vi "PDF Standard Kopf IAGnG.vi"(4 "L!L2 Cluster":T2, 5 "Gaschflasche Cluster":T3, 6 "Oprtionen Cluster":T5, 7 "Gas Komponente":cluster{"Komponente:":T4, "Konzentration":dbl} {"Konzentration" format="%#.6f"}, 8 "error in (no error)":errorcluster caption="Fehler (Eingang, kein Fehler)", 9 "LIN Pototokoll-Cluster (opotional)":T6 {"zusätzliche Zeitdauer Erster Punkt" format="%#_5g"; "Lin Modus" items=["Cal Gas to PNS", "Cal Gas to Samplepoint", "Measure"]; "Gas Ablaufdatum" format="%<%d.%m.%Y>T"; "HovaCAL Flow AutoLin"."HovaCAL Flow Input Cluster" format="%.2f"; "Gasflasche" items=["----"=10000, "IAG MG"=0, "IAG NH3 3000"=1, "IAG NH3 2000"=2, "IAG NH3 200"=3]; "Conditions:" items=["field", "laboratory"]; "Kalibrierauswahl" items=["Inaktiv", "Aktiv"]; "Anzahl Stufen" format="%#_5g"; "Zeitdauer Stufe" format="%#_5g"; "Verdünnungsgas" items=["N2", "O2"]; "Komponentenauswahl"."Konzentration" format="%#.6f"; "Gasnummer:" min=1 max=5; "Prüfgas Konzentration" format="%#.6f"; "Polynomkoeff." format="%#_18f"}, 10 "Analysator":string, 11 "Bearbeiter/in":string) -> (0 "error out":errorcluster caption="Fehler (Ausgang)", 1 "Header Size":i32, 2 "Header Values":T1[](array[typedef]), 3 "Header Labels":string[](array[string]))   [LabVIEW 2020, in "PDF Interface.lvlib"]
uses:
  PDF Interface.lvlib
  Linearisierung V2/Lin-Polynom Daten.ctl
  Linearisierung V2/KomponentenArray.ctl
  Visualisierungs Elemente/Auswahlfeld.ctl
  Visualisierungs Elemente/Zahlen-Eingabefeld.ctl
  Linearisierung V2/EPA Optionsfeld.ctl
  Linearisierung V2/Gasteiler/HovaCal/AutoLin Hovacal.ctl
  Linearisierung V2/Kalibrieroption.ctl
  Linearisierung V2/EPA1065-307/Condition.ctl
  Seiten/System Einstellungen V2/Konfig Gasflasche.ctl
  Seiten/System Einstellungen V2/Gasflasche Auswahl.ctl
  Linearisierung V2/Gasteiler/HovaCAL_Interface/Controls/Flow Einstellung.ctl
  Linearisierung V2/Gasteiler/HovaCAL_Interface/Controls/Pump state.ctl
  Seiten/CalGas Aufschaltung/Lin Modus.ctl
  PDF Protokoll Standard Kopf Optionen.ctl
  Visualisierungs Elemente/String - Ausgabefeld.ctl
  PDF Protokoll Standard Kopf Gasflasche Auswahl.ctl
  Seiten/System Einstellungen V2/Aktioen FGV System Konstanten.ctl
  Seiten/System Einstellungen V2/Aktion FGV SystemEinstellungenV2.ctl
  Sprachverwaltung/FGV Aktion Tabelle zerlegen.ctl
  Seiten/System Einstellungen V2/System Einstellungen V2.lvlib
  Sprachverwaltung/Sprachverwaltung.lvlib
  Seiten/Gaszuordnung AO/Gaszuordnung AO.lvlib
  Linearisierung V2/Linearisierung v2.lvlib
  Linearisierung V2/Gasteiler/Gasteiler.lvlib
  Linearisierung V2/Gasteiler/HovaCal/HovaCal.lvlib
  Linearisierung V2/EPA1065-307/Linearity verification 1065-307.lvlib
  Linearisierung V2/Gasteiler/HovaCAL_Interface/Controls/Controls.lvlib
  Seiten/CalGas Aufschaltung/CalGas Aufschaltung.lvlib
panel:
  # "%"
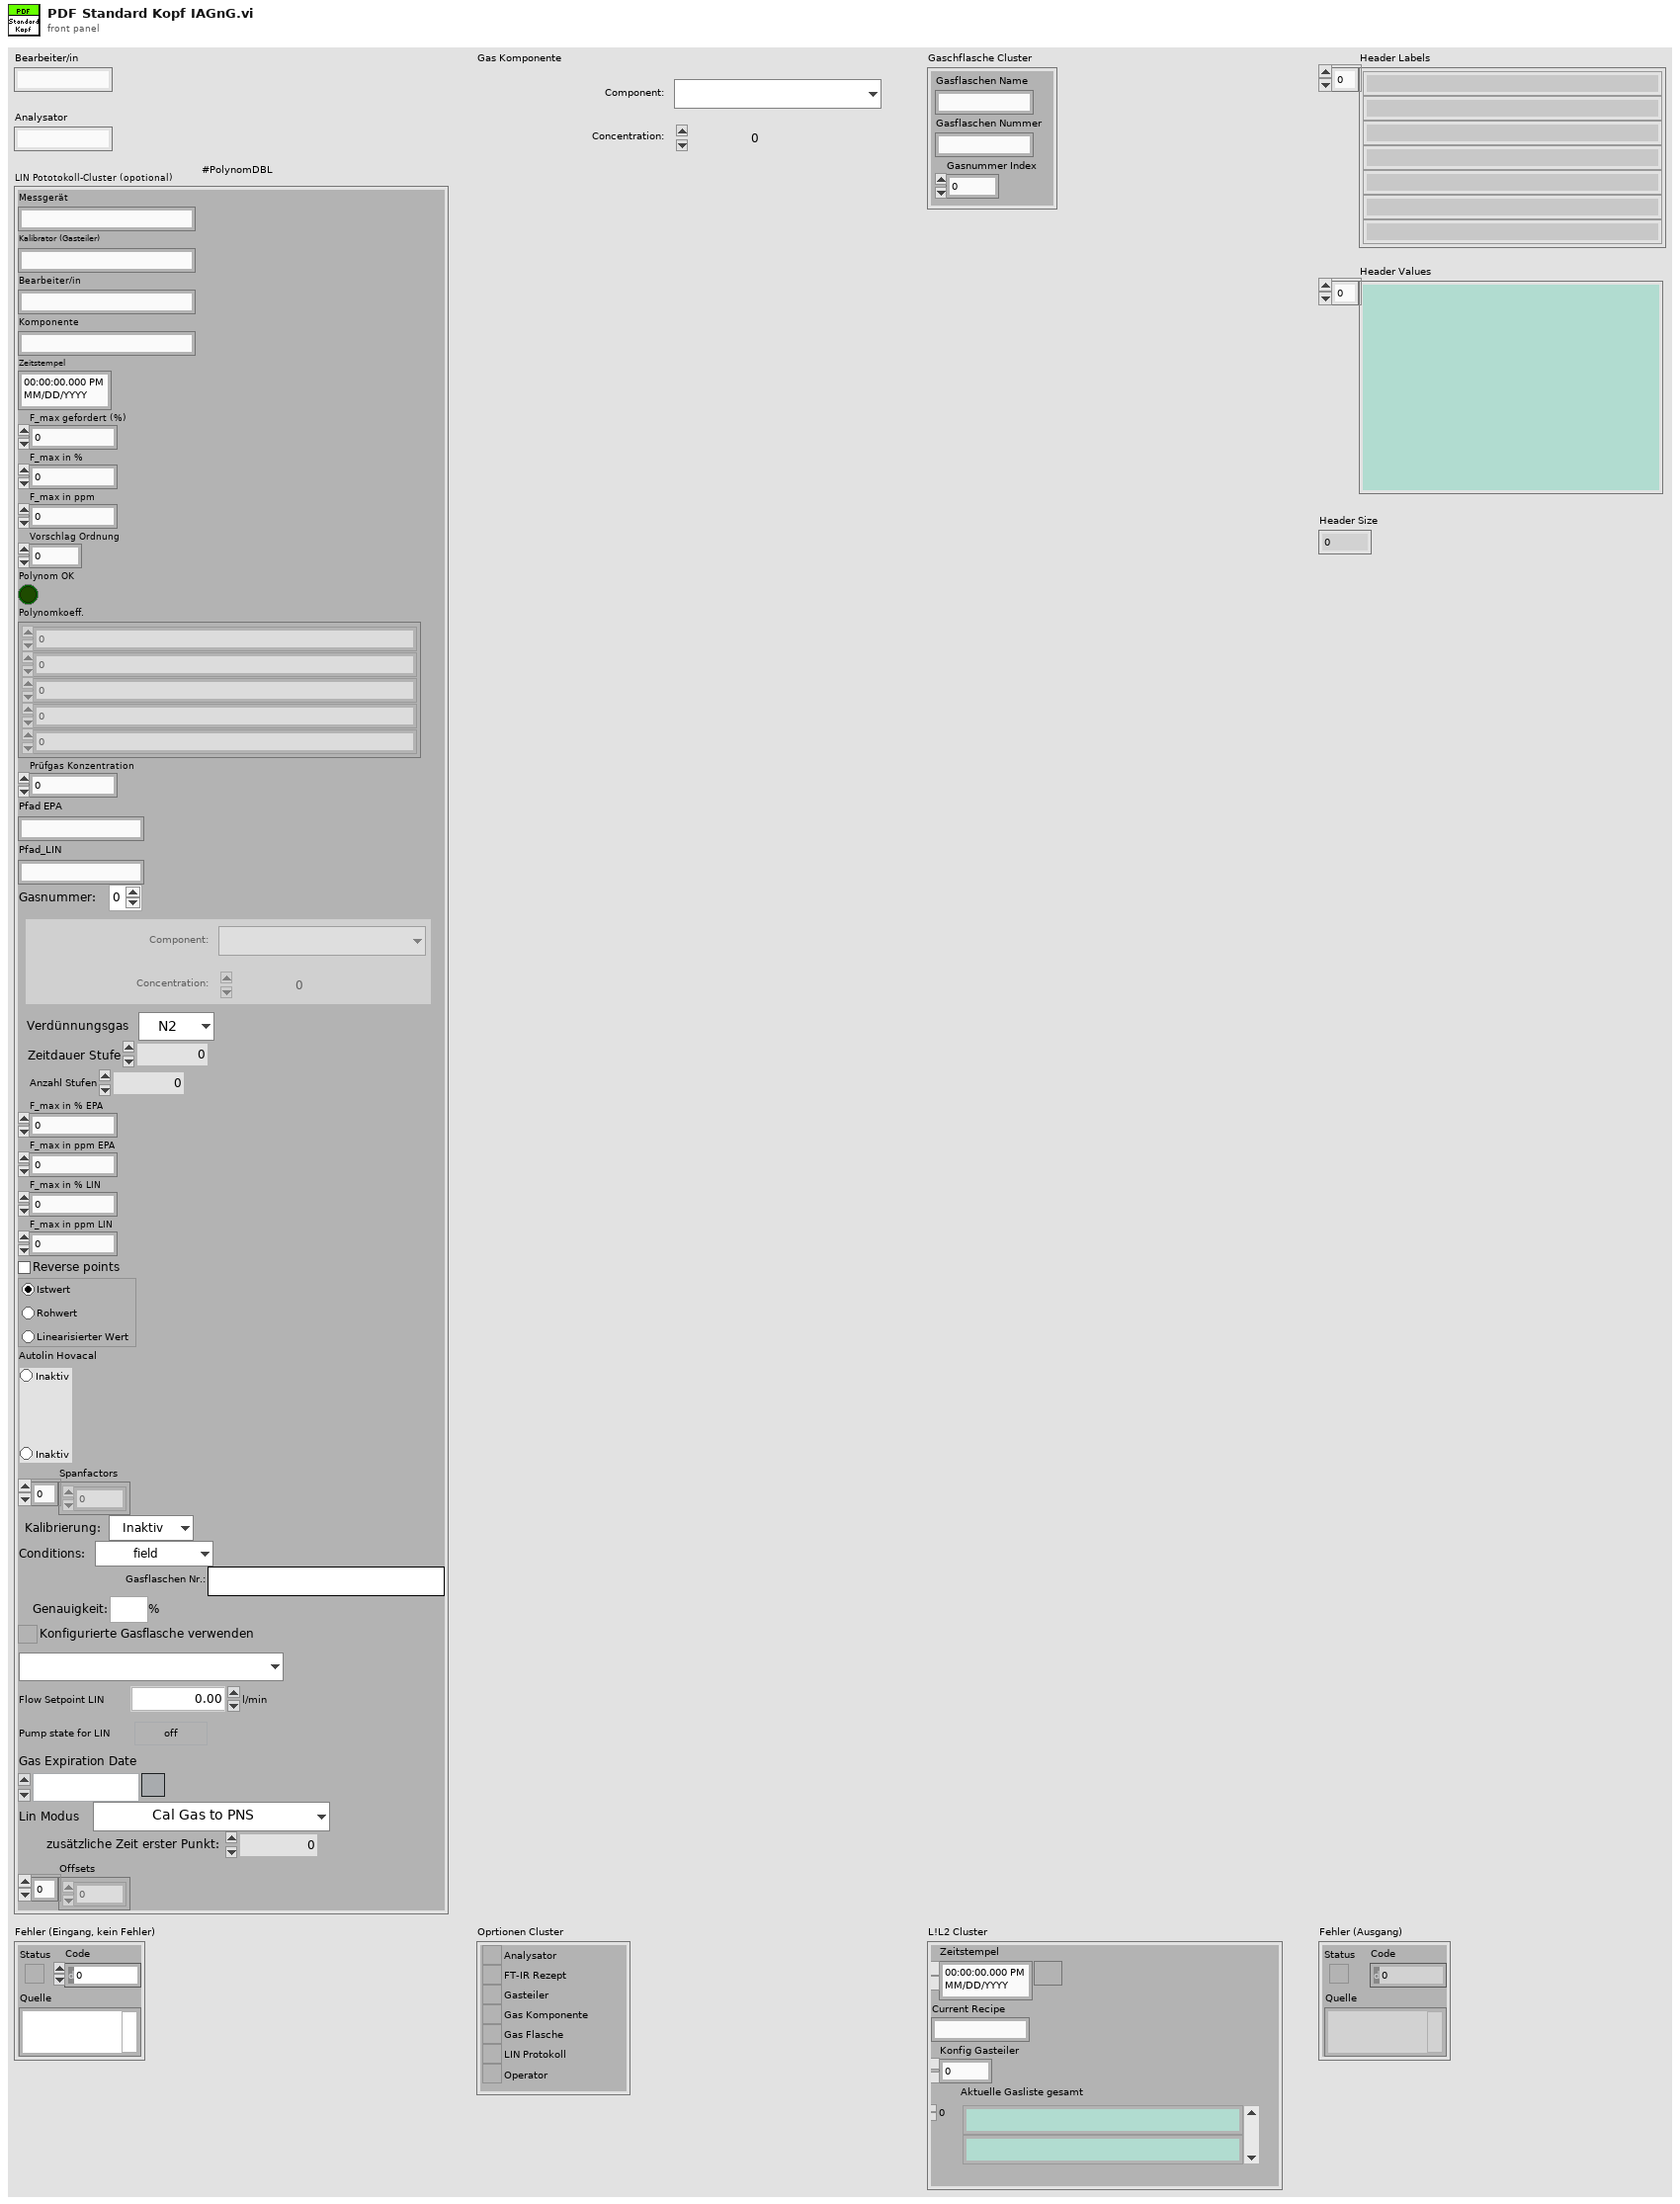
[diagram p1: front panel]
types:
  T1 = typedef "String - Ausgabefeld.ctl" = string
  T2 = cluster{"Zeitstempel":timestamp, "Current Recipe":string, "Konfig Gasteiler":i32, "Aktuelle Gasliste gesamt":T1[]}
  T3 = typedef "PDF Interface.lvlib/PDF Protokoll Standard Kopf Gasflasche Auswahl.ctl" = cluster{"Gasflaschen Name":string, "Gasflaschen Nummer":string, "Gasnummer Index":i32}
  T4 = typedef "Auswahlfeld.ctl" = u16
  T5 = typedef "PDF Interface.lvlib/PDF Protokoll Standard Kopf Optionen.ctl" = cluster{"Analysator":bool, "FT-IR Rezept":bool, "Gasteiler":bool, "Gas Komponente":bool, "Gas Flasche":bool, "LIN Protokoll":bool, "Operator":bool}
  T6 = typedef "Linearisierung v2.lvlib/Lin-Polynom Daten.ctl" = cluster{"Messgerät":string, "Kalibrator (Gasteiler)":string, "Bearbeiter/in":string, "Komponente":string, "Zeitstempel":timestamp, "F_max gefordert (%)":sgl, "F_max in %":sgl, "F_max in ppm":sgl, "Vorschlag Ordnung":i32, "Polynom OK":bool, "Polynomkoeff.":dbl[], "Prüfgas Konzentration":dbl, "Pfad EPA":string, "Pfad_LIN":string, "Gasnummer:":u8, "Komponentenauswahl":T7, "Verdünnungsgas":T8, "Zeitdauer Stufe":T9, "Anzahl Stufen":T9, "F_max in % EPA":sgl, "F_max in ppm EPA":sgl, "F_max in % LIN":sgl, "F_max in ppm LIN":sgl, "Punkte umkehren":bool, "EPA Optionsfeld":T10, "Autolin Hovacal":T11, "Spanfactors":sgl[], "Kalibrierauswahl":T12, "Conditions:":T13, "Gasflaschen Nr.:":string, "Bottle Accuracy":dbl, "Konfig Gasflasche":T14, "Gasflasche":T15, "HovaCAL Flow AutoLin":T16, "MFC Output":T17, "Gas Ablaufdatum":timestamp, "Lin Modus":T18, "zusätzliche Zeitdauer Erster Punkt":sgl, "Offsets":sgl[]}
  T7 = typedef "Linearisierung v2.lvlib/KomponentenArray.ctl" = cluster{"Komponente:":T4, "Konzentration":dbl}[]
  T8 = typedef "Linearisierung v2.lvlib/Gasteiler.lvlib/Prüfgas in.ctl" = u16
  T9 = typedef "Zahlen-Eingabefeld.ctl" = sgl
  T10 = typedef "Linearisierung v2.lvlib/EPA Optionsfeld.ctl" = enum32{"Istwert", "Rohwert", "Linearisierter Wert"}
  T11 = typedef "Linearisierung v2.lvlib/Gasteiler.lvlib/HovaCal.lvlib/AutoLin Hovacal.ctl" = enum32{"Keine Auswahl", "Optionsauswahl 1", "Optionsauswahl 2"}
  T12 = typedef "Linearisierung v2.lvlib/Kalibrieroption.ctl" = u16
  T13 = typedef "Linearisierung v2.lvlib/Linearity verification 1065-307.lvlib/Condition.ctl" = u16
  T14 = typedef "System Einstellungen V2.lvlib/Konfig Gasflasche.ctl" = bool
  T15 = typedef "System Einstellungen V2.lvlib/Gasflasche Auswahl.ctl" = u16
  T16 = typedef "Linearisierung v2.lvlib/Gasteiler.lvlib/HovaCAL_Interface.lvlib/Controls.lvlib/Flow Einstellung.ctl" = cluster{"HovaCAL Flow Input Cluster":dbl}
  T17 = typedef "Linearisierung v2.lvlib/Gasteiler.lvlib/HovaCAL_Interface.lvlib/Controls.lvlib/Pump state.ctl" = cluster{"Run":bool}
  T18 = typedef "CalGas Aufschaltung.lvlib/Lin Modus.ctl" = u16
  T19 = typedef "Sprachverwaltung.lvlib/FGV Aktion Tabelle zerlegen.ctl" = enum16{"laden", "vereinzeln", "speichern"}
  T20 = typedef "System Einstellungen V2.lvlib/Aktion FGV SystemEinstellungenV2.ctl" = enum16{"lesen", "Analysatoren schreiben", "Analysator ändern", "Analysatoren löschen", "laden", "speichern", "Untertitel", "Analysatoren", "Neue Analysatoren", "Gasteiler schreiben", "Gasteiler ändern", "Gasteiler löschen", "Gasteiler", "Gasteiler exportieren", "Gasteiler importieren"}
  T21 = typedef "System Einstellungen V2.lvlib/Aktioen FGV System Konstanten.ctl" = enum16{"lesen", "laden", "speichern", "Sprache"}
  T22 = typedef "System Einstellungen V2.lvlib/Gasteiler.ctl" = cluster{"Gasteiler Name":string, "Gasteiler Type":string, "Gasteiler Seriennummer":string, "Gasteiler Letzte Wartung":timestamp}
  T23 = cluster{"GasteilerDefinitionsListe":T22[], "GasteilerDefinitionTextliste":string[][], "Gasteiler Strings And Values":cluster{"String":string, "Wert":string}[]}
  T24 = typedef "System Einstellungen V2.lvlib/Traegergas.ctl" = string
  T25 = cluster{"Modell":string, "ProjektNummer":string, "Software Version":string, "Seriennummer":string}
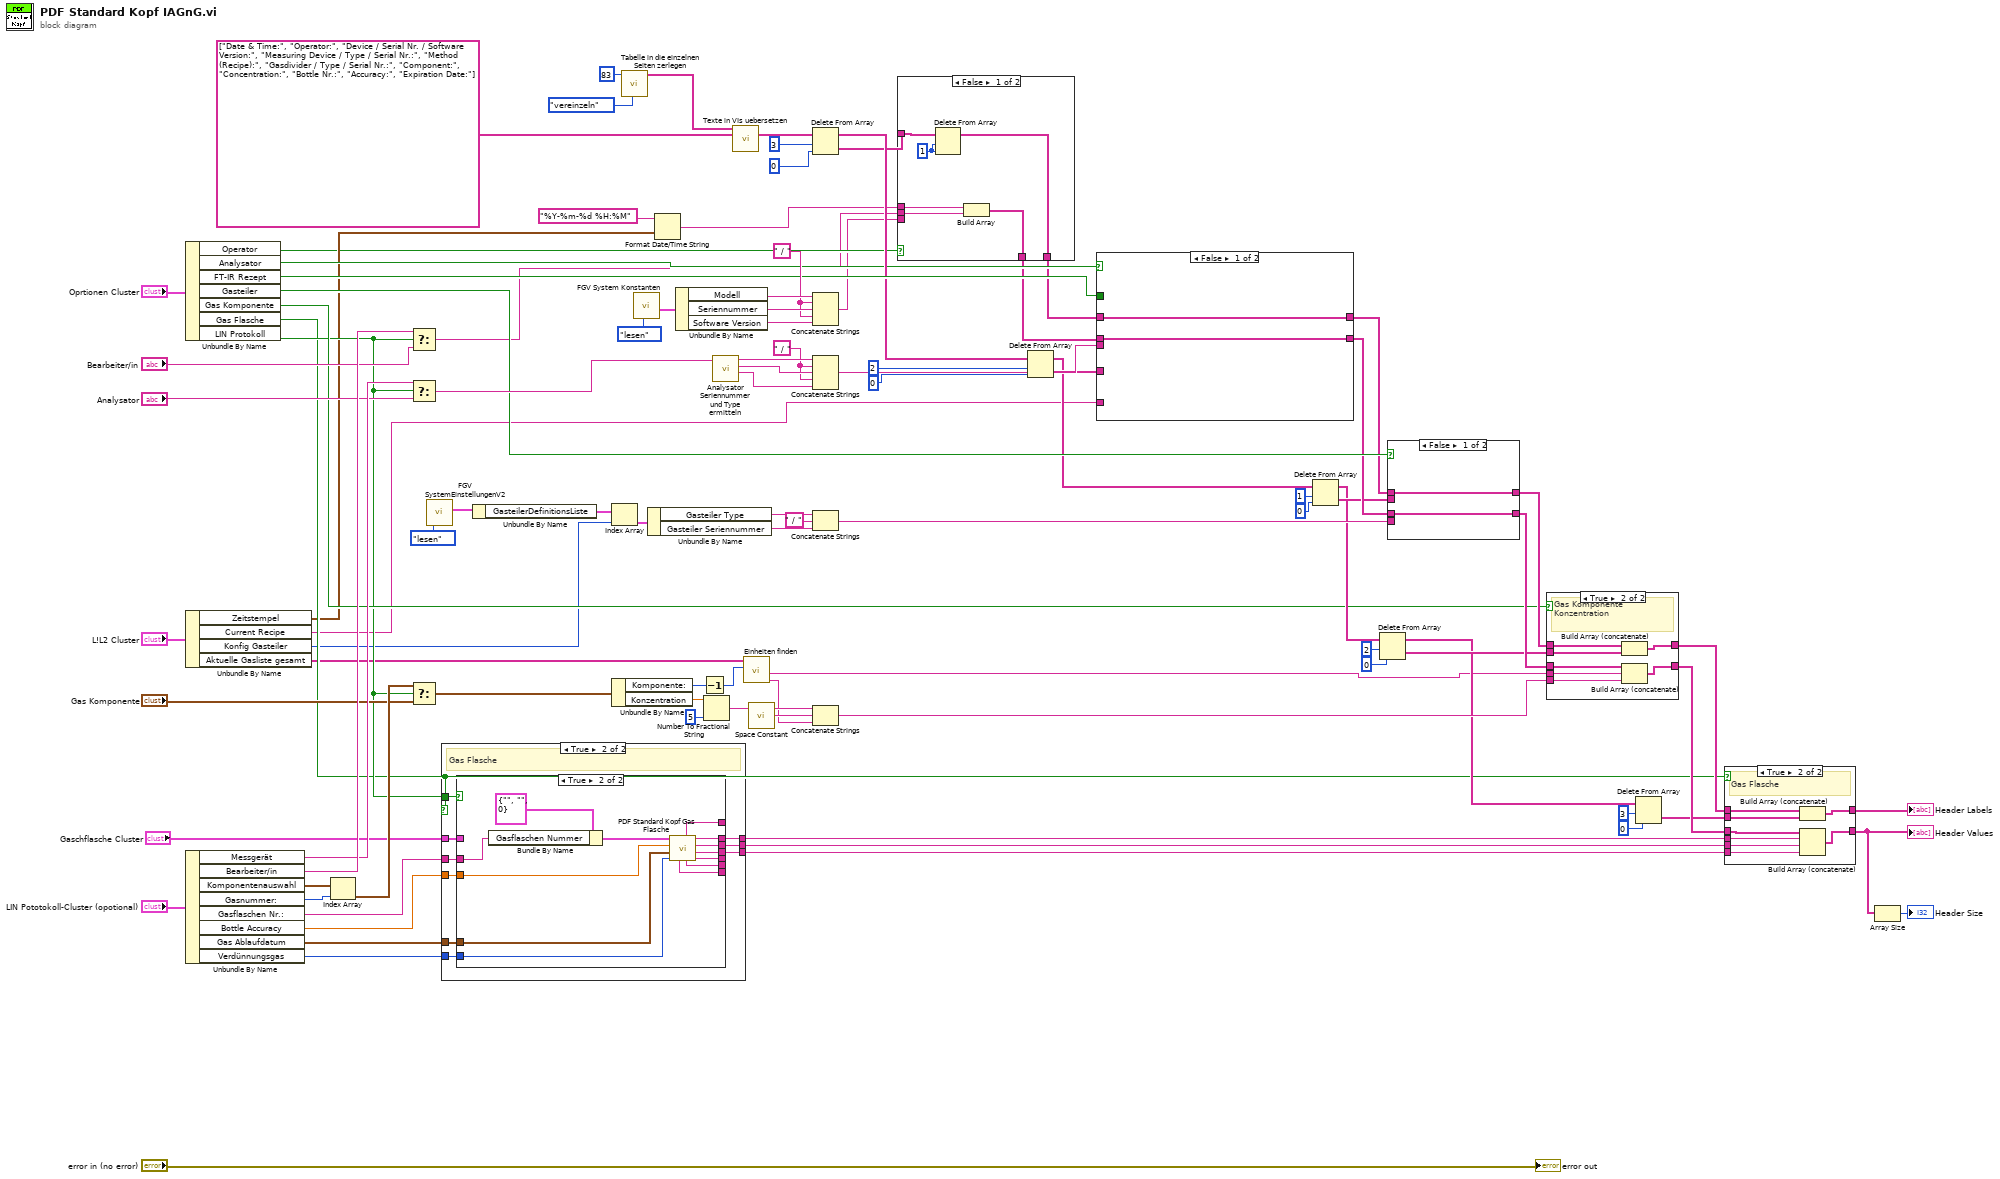
[diagram p0: block diagram]
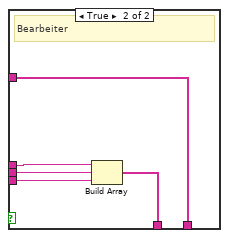
[diagram p2: hidden frame]
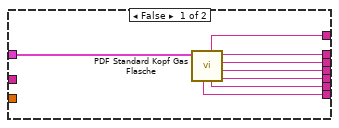
[diagram p5: hidden frame]
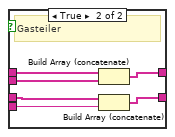
[diagram p7: hidden frame]
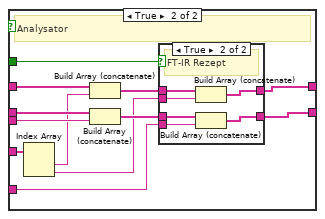
[diagram p8: hidden frame]
diagram:
  w80 = " / " ("String")
  w77 = " / " ("String")
  n1 = Unbundle By Name("Oprtionen Cluster") -> ("Operator"=w7:bool, "Analysator"=w57:bool, "FT-IR Rezept"=w63:bool, "Gasteiler"=w56:bool, "Gas Komponente"=w37:bool, "Gas Flasche"=w26:bool, "LIN Protokoll"=w36:bool)
  n2 = Unbundle By Name("L!L2 Cluster") -> ("Zeitstempel"=w10:timestamp, "Current Recipe"=w9:string, "Konfig Gasteiler"=w8:i32, "Aktuelle Gasliste gesamt"=w11:T1[])
  n3 = Unbundle By Name("LIN Pototokoll-Cluster (opotional)") -> ("Messgerät"=w66:string, "Bearbeiter/in"=w68:string, "Komponentenauswahl"=w88:T7, "Gasnummer:"=w87:u8, "Gasflaschen Nr.:"=w35:string, "Bottle Accuracy"=w34:dbl, "Gas Ablaufdatum"=w19:timestamp, "Verdünnungsgas"=w18:T8)
  n4 = Index Array(array=w88, index=w87) -> (element=w41:cluster{"Komponente:":T4, "Konzentration":dbl})
  n5 = Select(t=w68, s=w36, f="Bearbeiter/in") -> (s? t:f=w3:string)
  n6 = Select(t=w66, s=w36, f="Analysator") -> (s? t:f=w64:string)
  n7 = Select(t=w41, s=w36, f="Gas Komponente") -> (s? t:f=w39:cluster{"Komponente:":T4, "Konzentration":dbl})
  n8 = call "FGV SystemEinstellungenV2.vi"("Aktion"=Aktion_FGV_SystemEinstellungenV2."lesen") -> ("Gasteiler"=w98:T23)  [unwired: 5 in, 5 out]
  n9 = case shown="True" w26 {
    tunnel: "Gaschflasche Cluster" -> [_ w109]
    tunnel: w36 -> [_ w108]
    tunnel: w35 -> [_ w107]
    tunnel: w34 -> [_ w106]
    tunnel: [_ w103] -> w20
    tunnel: [_ w105] -> w27
    tunnel: [_ w104] -> w21
    tunnel: w19 -> [_ w102]
    tunnel: w18 -> [_ w101]
    frame False {
    }
    frame True {
      # "Gas Flasche"
      n10 = case shown="True" w108 {
        tunnel: w109 -> [w117 _]
        tunnel: w107 -> [_ w129]
        tunnel: w106 -> [_ w120]
        tunnel: [w116 w127] -> w105
        tunnel: [w115 w126] -> w104
        tunnel: [w114 w125] -> w103
        tunnel: [w113 w124] -> _
        tunnel: [w112 w123] -> _
        tunnel: [w111 w122] -> _
        tunnel: [w110 w121] -> _
        tunnel: w102 -> [_ w119]
        tunnel: w101 -> [_ w118]
        frame False {
          n11 = call "PDF Standard Kopf Gas Flasche.vi"("Gaschflasche Auswahl Cluster"=w117) -> ("Konzentration"=w112:string, "Ablaufdatum"=w114:string, "Genauigkeit"=w115:string, "Chargennummer"=w116:string, "Gasauswahl"=w111:string, "Gasname für die Auswahl"=w113:string, "Trägergas"=w110:T24)  [unwired: 4 in]
        }
        frame True {
          n12 = Bundle By Name(cluster=T3 {"Gasflaschen Name"="", "Gasflaschen Nummer"="", "Gasnummer Index"=0} ("Gaschflasche Auswahl Cluster"), "Gasflaschen Nummer"=w129) -> (w128:T3)
          n13 = call "PDF Standard Kopf Gas Flasche.vi"("Verdünnungsgas"=w118, "Ablaufdatum"=w119, "Genauigkeit in"=w120, "Gaschflasche Auswahl Cluster"=w128) -> ("Konzentration"=w123:string, "Ablaufdatum"=w125:string, "Genauigkeit"=w126:string, "Chargennummer"=w127:string, "Gasauswahl"=w122:string, "Gasname für die Auswahl"=w124:string, "Trägergas"=w121:T24)  [unwired: 1 in]
        }
      }
    }
  }
  n14 = Unbundle By Name(w98) -> ("GasteilerDefinitionsListe"=w97:T22[])
  n15 = Index Array(array=w97, index=w8) -> (element=w96:T22)
  n16 = Unbundle By Name(w39) -> ("Komponente:"=w84:T4, "Konzentration"=w86:dbl)
  n17 = call "Tabelle in die einzelnen Seiten zerlegen.vi"("Aktion"=FGV_Aktion_Tabelle_zerlegen."vereinzeln", "Index (Seite)"=83) -> ("Sprachliste"=w74:string[][])  [unwired: 7 in, 2 out]
  n18 = call "FGV System Konstanten.vi"("Aktionen"=Aktioen_FGV_System_Konstanten."lesen") -> ("Cluster out"=w100:T25)  [unwired: 6 in, 4 out]
  n19 = Unbundle By Name(w96) -> ("Gasteiler Type"=w92:string, "Gasteiler Seriennummer"=w91:string)
  n20 = Format Date/Time String(time format string (%c)="%Y-%m-%d %H:%M" ("Zeitformatierungs-String (%c)"), seconds (now)=w10) -> (date/time string=w4:string)  [unwired: 1 in]
  n21 = Unbundle By Name(w100) -> ("Modell"=w95:string, "Seriennummer"=w94:string, "Software Version"=w78:string)
  n22 = Decrement(x=w84) -> (x-1=w14:T4)
  n23 = Number To Fractional String(number=w86, precision (6)=i16 5 ("Genauigkeit (6)")) -> (F-format string=w83:string)  [unwired: 2 in]
  n24 = call "Analysator Seriennummer und Type ermitteln.vi"("Analysator"=w64) -> ("Seriennummer"=w81:string, "Type"=w89:string, "Name für Protokoll"=w90:string)  [unwired: 8 in]
  n25 = call "Texte in VIs uebersetzen.vi"("Sprachliste"=w74, "String-Array zum Übersetzen"=string[] ["Date & Time:", "Operator:", "Device / Serial Nr. / Software Version:", "Measuring Device / Type / Serial Nr.:", "Method (Recipe):", "Gasdivider / Type / Serial Nr.:", "Component:", "Concentration:", "Bottle Nr.:", "Accuracy:", "Expiration Date:"]) -> ("String-Array zum Übersetzen"=w71:string[])  [unwired: 9 in, 4 out]
  n26 = call "Einheiten finden.vi"("Komponente"=w14, "Aktuelle Gasliste gesamt"=w11) -> ("Einheit in String"=w13:string, "Komponenten Name"=w15:T1)  [unwired: 8 in]
  n27 = call <vilib>:"Space Constant.vi"() -> ("String"=w82:string)
  n28 = Delete From Array(array=w71, length=3 ("Länge"), index=0 ("Index")) -> (deleted portion=w6:string[], array with subset deleted=w61:string[])
  n29 = Concatenate Strings(w95, w77, w94, w77, w78) -> (w2:string)
  n30 = Concatenate Strings(w90, w80, w89, w80, w81) -> (w62:string)
  n31 = Concatenate Strings(w92, " / " ("String"), w91) -> (w55:string)
  n32 = Concatenate Strings(w83, w82, w13) -> (w38:string)
  n33 = case shown="False" w7 {
    tunnel: w6 -> [w136 w141]
    tunnel: [w134 w141] -> w5
    tunnel: w4 -> [w133 w140]
    tunnel: w3 -> [_ w139]
    tunnel: w2 -> [w132 w138]
    tunnel: [w131 w137] -> w1
    frame False {
      w135 = 1 ("Index")
      n34 = Delete From Array(array=w136, length=w135, index=w135) -> (array with subset deleted=w134:string[])  [unwired: 1 out]
      n35 = Build Array(w133, w132) -> (w131:string[])
    }
    frame True {
      # "Bearbeiter"
      n36 = Build Array(w140, w139, w138) -> (w137:string[])
    }
  }
  n37 = Delete From Array(array=w61, length=2 ("Länge"), index=0 ("Index")) -> (deleted portion=w58:string[], array with subset deleted=w50:string[])
  n38 = case shown="False" w57 {
    tunnel: w5 -> [w143 w155]
    tunnel: w1 -> [w142 w154]
    tunnel: w63 -> [_ w153]
    tunnel: w62 -> [_ w152]
    tunnel: w58 -> [_ w151]
    tunnel: [w143 w148] -> w54
    tunnel: [w142 w147] -> w53
    tunnel: w9 -> [_ w146]
    frame False {
    }
    frame True {
      # "Analysator"
      n39 = Index Array(array=w151) -> (element #1=w145:string, element #2=w144:string)  [unwired: 2 in]
      n40 = Build Array (concatenate)(w155, w145) -> (w150:string[])
      n41 = Build Array (concatenate)(w154, w152) -> (w149:string[])
      n42 = case shown="True" w153 {
        tunnel: w150 -> [w157 w163]
        tunnel: w149 -> [w156 w162]
        tunnel: [w157 w161] -> w148
        tunnel: [w156 w160] -> w147
        tunnel: w146 -> [_ w159]
        tunnel: w144 -> [_ w158]
        frame False {
        }
        frame True {
          # "FT-IR Rezept"
          n43 = Build Array (concatenate)(w163, w158) -> (w161:string[])
          n44 = Build Array (concatenate)(w162, w159) -> (w160:string[])
        }
      }
    }
  }
  n45 = Delete From Array(array=w50, length=1 ("Länge"), index=0 ("Index")) -> (deleted portion=w49:string[], array with subset deleted=w42:string[])
  n46 = Delete From Array(array=w42, length=2 ("Länge"), index=0 ("Index")) -> (deleted portion=w43:string[], array with subset deleted=w29:string[])
  n47 = case shown="False" w56 {
    tunnel: w55 -> [_ w171]
    tunnel: w54 -> [w165 w170]
    tunnel: w53 -> [w164 w169]
    tunnel: [w165 w168] -> w47
    tunnel: [w164 w167] -> w46
    tunnel: w49 -> [_ w166]
    frame False {
    }
    frame True {
      # "Gasteiler"
      n48 = Build Array (concatenate)(w170, w166) -> (w168:string[])
      n49 = Build Array (concatenate)(w169, w171) -> (w167:string[])
    }
  }
  n50 = case shown="True" w37 {
    tunnel: w15 -> [_ w174]
    tunnel: w47 -> [w173 w180]
    tunnel: w46 -> [w172 w176]
    tunnel: [w173 w179] -> w33
    tunnel: [w172 w178] -> w32
    tunnel: w43 -> [_ w177]
    tunnel: w38 -> [_ w175]
    frame False {
    }
    frame True {
      # "Gas Komponente\nKonzentration"
      n51 = Build Array (concatenate)(w180, w177) -> (w179:string[])
      n52 = Build Array (concatenate)(w176, w174, w175) -> (w178:T1[])
    }
  }
  n53 = Delete From Array(array=w29, length=3 ("Länge"), index=0 ("Index")) -> (deleted portion=w28:string[])  [unwired: 1 out]
  n54 = case shown="True" w26 {
    tunnel: w27 -> [_ w190]
    tunnel: w33 -> [w182 w189]
    tunnel: w32 -> [w181 w188]
    tunnel: [w182 w187] -> w25
    tunnel: [w181 w186] -> w24
    tunnel: w28 -> [_ w185]
    tunnel: w21 -> [_ w184]
    tunnel: w20 -> [_ w183]
    frame False {
    }
    frame True {
      # "Gas Flasche"
      n55 = Build Array (concatenate)(w189, w185) -> (w187:string[])
      n56 = Build Array (concatenate)(w188, w190, w184, w183) -> (w186:T1[])
    }
  }
  "Header Labels" <- w25
  "Header Values" <- w24
  n57 = Array Size(array=w24) -> (size(s)=→"Header Size":i32)
  "error out" <- "error in (no error)"
